vi "Periodic Tasks.vi"(8 "error in":errorcluster) -> ()   [LabVIEW 2017]
doc: "This VI runs in parallel to other tasks. It can contain as many user-defined periodic loops as you need. These can carry out PID or other sorts of timed response."
uses:
  Motor Enums.ctl
  Robot Global Data.vi
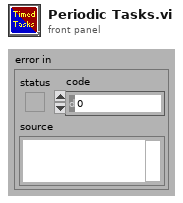
[diagram p1: front panel]
types:
  T1 = typedef "Motor Enums.ctl" = enum16{"drive joystick", "arm joystick", "left motor", "right motor", "elevator", "lever", "claw"}
  T2 = typedef "WPI_MotorControlDeviceRef.ctl" = cluster{"DeviceStatus":errorcluster, "Type":T3, "PWM":cluster{"PWM Channel":T4, "DeadBand":T5}, "CAN":cluster{"Device Number":u8, "SetOutput VI Ref":variant, "GetOutput VI Ref":variant, "Enable VI Ref":variant, "Disable VI Ref":variant, "Data":variant}, "Invert":bool, "DIO PWM":cluster{"PWM \"Enable\" Channel":T4, "DIOChannel":T6, "PWM Rate":dbl}}
  T3 = typedef "WPI_MotorControlType.ctl" = enum16{"PWM", "CAN", "DIO PWM"}
  T4 = typedef "FPGA_DIOPWMChannel.ctl" = enum8{"PWM 0", "PWM 1", "PWM 2", "PWM 3", "PWM 4", "PWM 5", "PWM 6", "PWM 7", "PWM 8", "PWM 9", "PWM MXP 0", "PWM MXP 1", "PWM MXP 2", "PWM MXP 3", "PWM MXP 4", "PWM MXP 5", "PWM MXP 6", "PWM MXP 7", "PWM MXP 8", "PWM MXP 9", "Invalid"}
  T5 = typedef "WPI_PWMDeadband.ctl" = cluster{"Name":string, "maxPositivePwm":i32, "minPositivePwm":i32, "centerPwm":i32, "maxNegativePwm":i32, "minNegativePwm":i32, "angularRange":u16}
  T6 = typedef "FPGA_DIOChannel.ctl" = enum8{"DIO 0", "DIO 1", "DIO 2", "DIO 3", "DIO 4", "DIO 5", "DIO 6", "DIO 7", "DIO 8", "DIO 9", "DIO MXP 0", "DIO MXP 1", "DIO MXP 2", "DIO MXP 3", "DIO MXP 4", "DIO MXP 5", "DIO MXP 6", "DIO MXP 7", "DIO MXP 8", "DIO MXP 9", "DIO MXP 10", "DIO MXP 11", "DIO MXP 12", "DIO MXP 13", "DIO MXP 14", "DIO MXP 15", "SPI Port CS1", "SPI Port CS2", "SPI Port CS3", "SPI Port MISO", "SPI Port MOSI", "Invalid"}
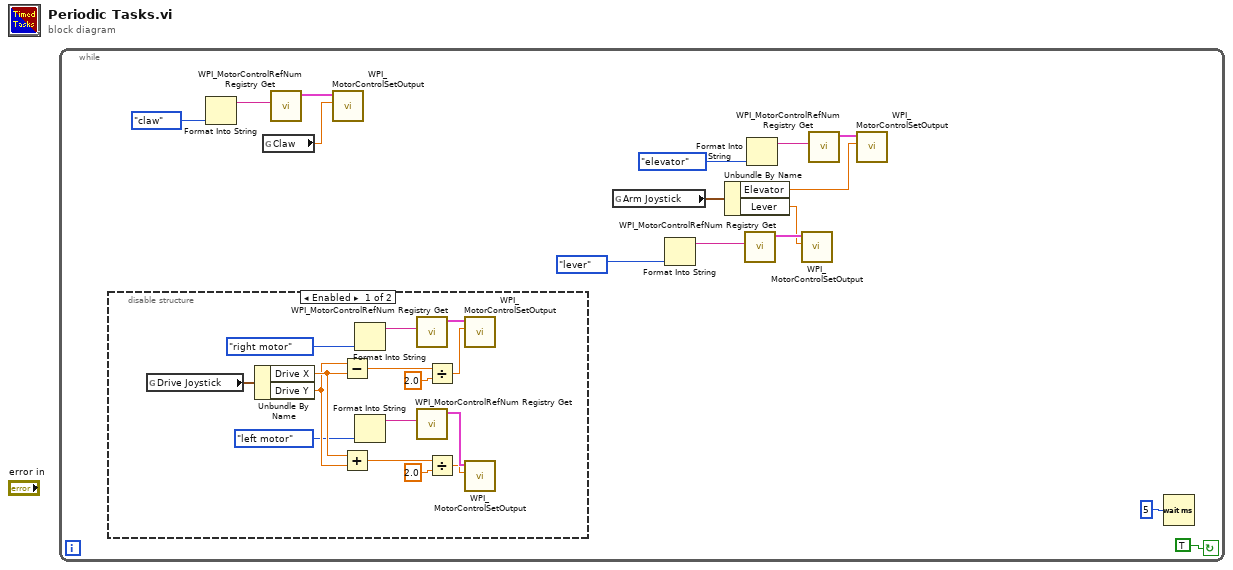
[diagram p0: block diagram]
diagram:
  n1 = while {
    stop <- TRUE continue-if-true
    n2 = disable-structure shown="Enabled" {
      frame Enabled {
        n3 = global read "Robot Global Data.vi" "Drive Joystick"() -> (w24:cluster{"Drive X":dbl, "Drive Y":dbl})
        n4 = Unbundle By Name(w24) -> ("Drive X"=w23:dbl, "Drive Y"=w22:dbl)
        n5 = Subtract(x=w22, y=w23) -> (x-y=w30:dbl)
        n6 = Add(x=w23, y=w22) -> (x+y=w29:dbl)
        n7 = Format Into String(Motor_Enums."right motor" ("Enum")) -> (resulting string=w16:string)  [unwired: 3 in, 1 out]
        n8 = Format Into String(Motor_Enums."left motor" ("Enum")) -> (resulting string=w18:string)  [unwired: 3 in, 1 out]
        n9 = call <vilib>:"WPI_MotorControlRefNum Registry Get.vi"("refnum name"=w16) -> ("MotorControlDevRef"=w26:T2)  [unwired: 9 in, 1 out]
        n10 = call <vilib>:"WPI_MotorControlRefNum Registry Get.vi"("refnum name"=w18) -> ("MotorControlDevRef"=w25:T2)  [unwired: 9 in, 1 out]
        n11 = Divide(x=w30, y=2.0) -> (x/y=w20:dbl)
        n12 = Divide(x=w29, y=2.0) -> (x/y=w21:dbl)
        n13 = call <vilib>:"WPI_MotorControlSetOutput.vi"("Output"=w20, "MotorControlDevRef"=w26) -> ()  [unwired: 7 in, 3 out]
        n14 = call <vilib>:"WPI_MotorControlSetOutput.vi"("Output"=w21, "MotorControlDevRef"=w25) -> ()  [unwired: 7 in, 3 out]
      }
      frame Disabled {
      }
    }
    n15 = Format Into String(Motor_Enums."claw" ("Enum")) -> (resulting string=w3:string)  [unwired: 3 in, 1 out]
    n16 = global read "Robot Global Data.vi" "Claw"() -> (w4:dbl)
    n17 = call <vilib>:"WPI_MotorControlRefNum Registry Get.vi"("refnum name"=w3) -> ("MotorControlDevRef"=w1:T2)  [unwired: 9 in, 1 out]
    n18 = call <vilib>:"WPI_MotorControlSetOutput.vi"("Output"=w4, "MotorControlDevRef"=w1) -> ()  [unwired: 7 in, 3 out]
    n19 = global read "Robot Global Data.vi" "Arm Joystick"() -> (w13:cluster{"Elevator":dbl, "Lever":dbl})
    n20 = Format Into String(Motor_Enums."lever" ("Enum")) -> (resulting string=w7:string)  [unwired: 3 in, 1 out]
    n21 = Unbundle By Name(w13) -> ("Elevator"=w12:dbl, "Lever"=w5:dbl)
    n22 = call <vilib>:"WPI_MotorControlRefNum Registry Get.vi"("refnum name"=w7) -> ("MotorControlDevRef"=w6:T2)  [unwired: 9 in, 1 out]
    n23 = Format Into String(Motor_Enums."elevator" ("Enum")) -> (resulting string=w10:string)  [unwired: 3 in, 1 out]
    n24 = call <vilib>:"WPI_MotorControlSetOutput.vi"("Output"=w5, "MotorControlDevRef"=w6) -> ()  [unwired: 7 in, 3 out]
    n25 = call <vilib>:"WPI_MotorControlRefNum Registry Get.vi"("refnum name"=w10) -> ("MotorControlDevRef"=w9:T2)  [unwired: 9 in, 1 out]
    n26 = call <vilib>:"WPI_MotorControlSetOutput.vi"("Output"=w12, "MotorControlDevRef"=w9) -> ()  [unwired: 7 in, 3 out]
    n27 = Wait (ms)(milliseconds to wait=u32 5) -> ()  [unwired: 1 out]
  }
